vi "RtdeAddInput.vi"(7 "RTDE Connect Parameters":refnum<k24>, 8 "Index for registers":i32, 9 "Data":i32(ring) items=["SpeedSliderMask", "SpeedSliderFraction", "StandardDigitalOutputMask", "ConfigurableDigitalOutputMask", "StandardDigitalOutput", "ConfigurableDigitalOutput", "StandardAnalogOutputMask", "StandardAnalogOutputType", "StandardAnalogOutput0", "StandardAnalogOutput1", "InputBtRegisters0To31", "InputBtRegisters32To63", "InputBitRegisters", "InputIntRegisters", "InputDoubleRegisters", "ExternalForceTorque"], 11 "error in":errorcluster) -> (3 "error out":errorcluster, 6 "RTDE Connect Parameters":refnum<k24>)   [LabVIEW 2024, in "UnderAutomation.UniversalRobots.lvlib"]
uses:
  UnderAutomation.UniversalRobots.lvlib
  C:/Users/fg/Documents/UniversalRobots.vi/LabVIEW_2024/UnderAutomation.UniversalRobots/lib/UnderAutomation.UniversalRobots.dll
  lib/UnderAutomation.UniversalRobots.dll
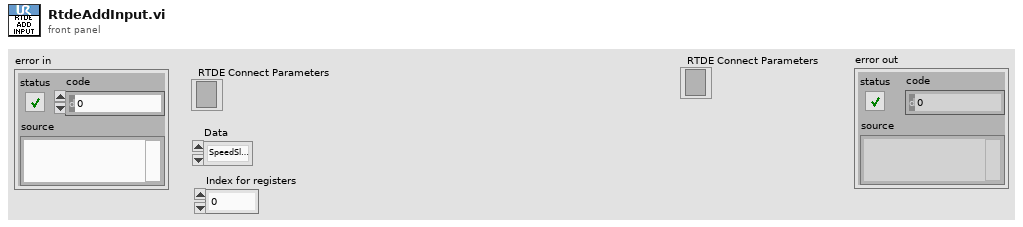
[diagram p1: front panel]
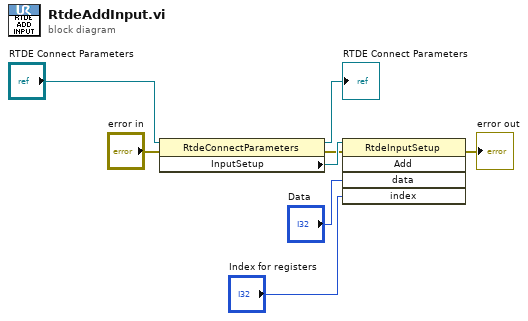
[diagram p0: block diagram]
diagram:
  n1 = property class="RtdeConnectParameters"(reference="RTDE Connect Parameters", error in="error in") -> (reference out=→"RTDE Connect Parameters":refnum<k24>, error out=w3:errorcluster, "InputSetup"=w7:refnum<k24>)
  n2 = invoke class="RtdeInputSetup" method="Add"(reference=w7, error in=w3, "data"="Data", "index"="Index for registers") -> (error out=→"error out":errorcluster)  [unwired: 1 in, 4 out]
